vi "SetInstrument name.vi"(0 "object in":refnum<class "KE2000.lvclass">, 1 "Instrument name":string, 5 "error in (no error)":errorcluster) -> (14 "object out":refnum<class "KE2000.lvclass">, 19 "error out":errorcluster)   [LabVIEW 2013, in "KE2000.lvclass"]
uses:
  KE2000.lvclass
  KE2000.lvclass/KE2000.ctl
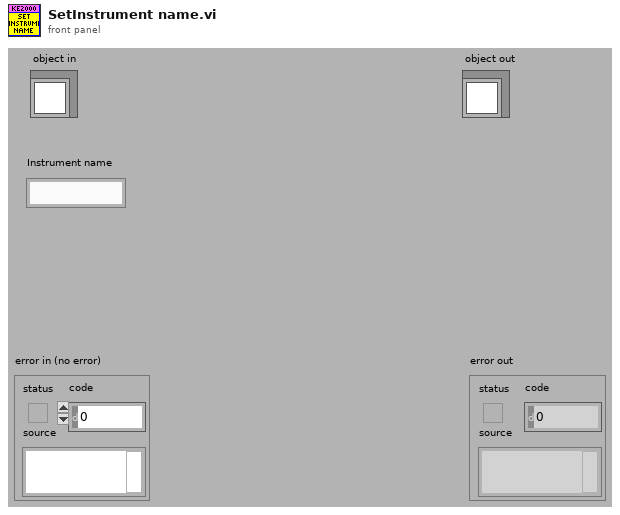
[diagram p1: front panel]
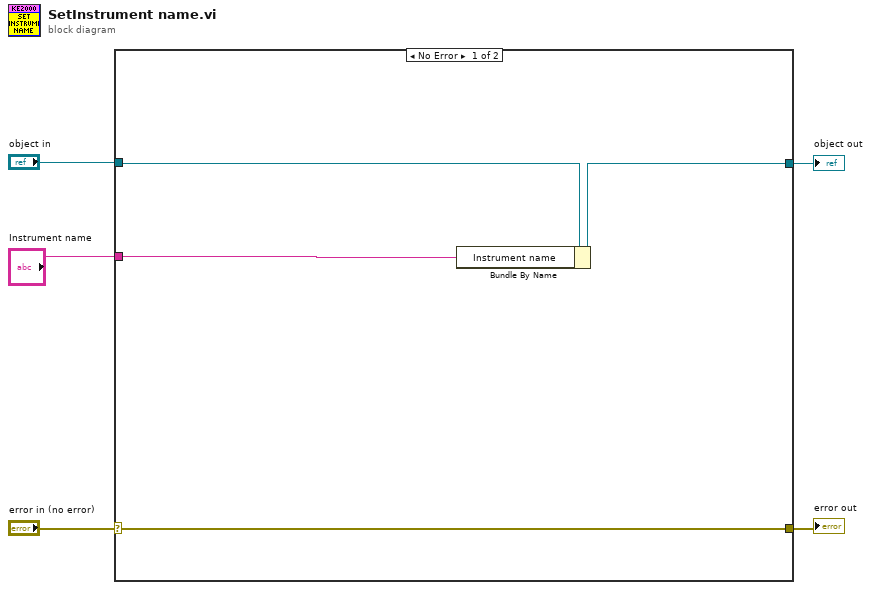
[diagram p0: block diagram]
diagram:
  n1 = case shown="No Error" "error in (no error)" {
    selector: "error in (no error)" -> [w8 w11]
    tunnel: [w8 w11] -> w4
    tunnel: [w6 w10] -> w2
    tunnel: "object in" -> [w7 w10]
    tunnel: "Instrument name" -> [w9 _]
    frame No Error {
      n2 = Bundle By Name(cluster=w7, "Instrument name"=w9) -> (w6:refnum<class "KE2000.lvclass">)
    }
    frame Error {
    }
  }
  "error out" <- w4
  "object out" <- w2
